vi "freqSet.vi"(4 "error in (no error)":errorcluster, 5 "SEQ in":u32, 6 "freq(MHz)":sgl, 7 "connection ID":refnum<k5>) -> (0 "error out":errorcluster, 1 "SEQ out":u32, 2 "OK？":bool, 3 "connection ID out":refnum<k5>)   [LabVIEW 2016]
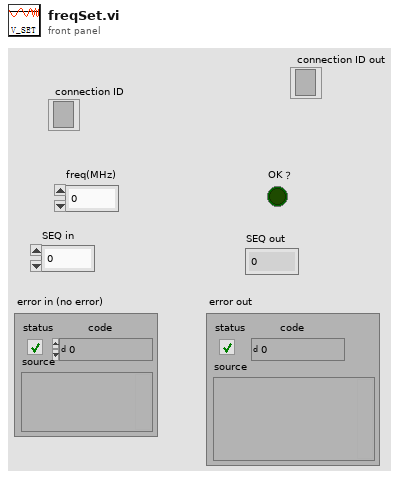
[diagram p1: front panel]
types:
  T1 = enum8{"SET_FREQ", "SET_VOLT", "SET_CHANNEL_VOLT", "SET_PHASE", "START_HEAT", "STOP_HEAT", "CHANNEL_CTRL_SINGLE", "CHANNEL_CTRL_ALL", "READ_VOLT_SET", "READ_VOLT_SET_RSP", "READ_CURRENT_VOLT", "READ_CURRENT_VOLT_RSP", "READ_PHASE", "READ_PHASE_RSP", "READ_HEATTIME_LEFT", "READ_HEATTIME_LEFT_RSP", "EXEC_RSP"}
  T2 = enum8{"SET_FREQ", "SET_VOLT", "SET_CHENNEL_VOLT", "SET_PHASE", "START_HEAT", "STOP_HEAT", "CHANNEL_CTRL_SINGLE", "CHANNEL_CTRL_ALL", "READ_VOLT_SET", "READ_VOLT_SET_RSP", "READ_CURRENT_VOLT", "READ_CURRENT_VOLT_RSP", "READ_PHASE", "READ_PHASE_RSP", "READ_HEATTIME_LEFT", "READ_HEATTIME_LEFT_RSP", "EXEC_RSP"}
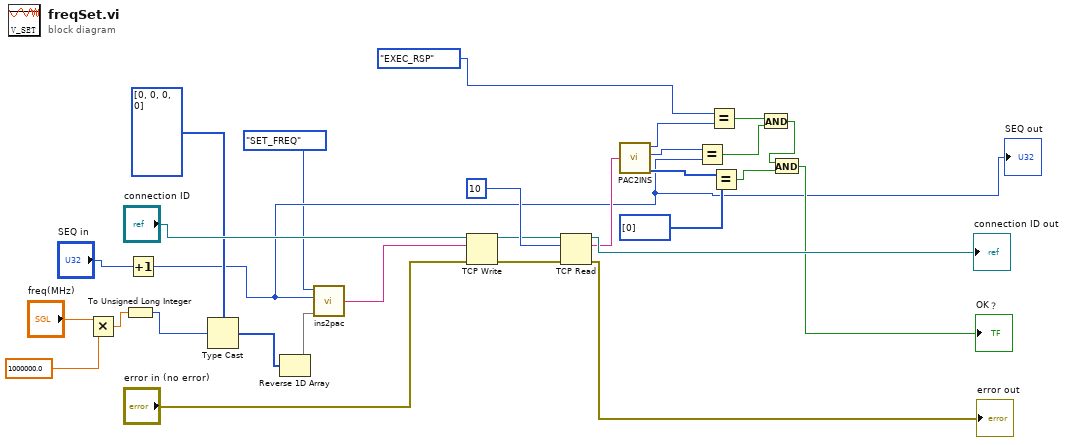
[diagram p0: block diagram]
diagram:
  n1 = Multiply(x="freq(MHz)", y=sgl 1000000.0) -> (x*y=w4:sgl)
  n2 = To Unsigned Long Integer(number=w4) -> (unsigned 32bit integer=w3:u32)
  n3 = Increment(x="SEQ in") -> (x+1=w10:u32)
  "SEQ out" <- w10
  n4 = Type Cast(type=u8[] [0, 0, 0, 0], x=w3) -> (*(type *) &x=w2:u8[])
  n5 = Reverse 1D Array(array=w2) -> (reversed array=w1:u8[])
  n6 = call "ins2pac.vi"("BODY"=w1, "SEQUENCE"=w10, "TYPE"=T1."SET_FREQ") -> ("PACKET"=w27:string)  [unwired: 1 in]
  n7 = TCP Write(connection ID="connection ID", data in=w27, error in (no error)="error in (no error)") -> (connection ID out=w24:refnum<k5>, error out=w23:errorcluster)  [unwired: 1 in, 1 out]
  n8 = TCP Read(connection ID=w24, bytes to read=10, error in (no error)=w23) -> (connection ID out=→"connection ID out":refnum<k5>, data out=w20:string, error out=→"error out":errorcluster)  [unwired: 2 in]
  n9 = call "PAC2INS.vi"("PACKET"=w20) -> ("TYPE"=w19:T2, "SEQUENCE"=w18:u32, "BODY"=w17:u8[])  [unwired: 1 out]
  n10 = Equal?(x=w18, y=w10) -> (x = y?=w14:bool)
  n11 = Equal?(x=T1."EXEC_RSP" ("TYPE"), y=w19) -> (x = y?=w15:bool)
  n12 = Equal?(x=w17, y=u8[] [0]) -> (x = y?=w12:bool)
  n13 = And(x=w15, y=w14) -> (x .and. y?=w13:bool)
  n14 = And(x=w13, y=w12) -> (x .and. y?=→"OK？":bool)
